vi "ke37xx Open Channels.vi"(0 "VISA Resource Name":refnum<visa-resource-name>, 1 "Channel List":string, 7 "Open All (False)":bool, 11 "error in (no error)":errorcluster) -> (4 "VISA Resource Name Out":refnum<visa-resource-name>, 15 "error out":errorcluster)   [LabVIEW 2009, in "Keithley 3700 Series.lvlib"]
doc: "This VI allows you to open a series of channels or to open all channels."
uses:
  <instrlib>/Keithley 3706/Keithley 3700 Series.lvlib
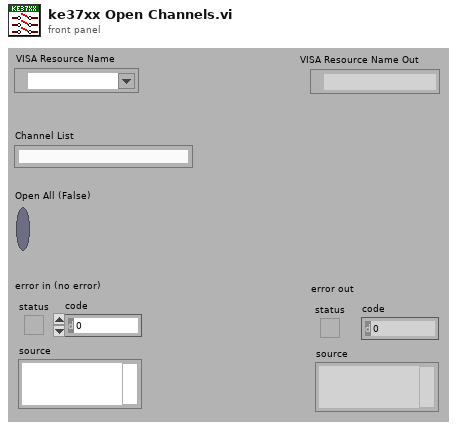
[diagram p1: front panel]
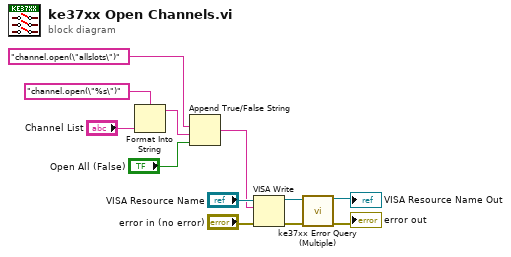
[diagram p0: block diagram]
diagram:
  n1 = Format Into String(format string="channel.open(\"%s\")", "Channel List") -> (resulting string=w2:string)  [unwired: 2 in, 1 out]
  n2 = Append True/False String(1:"Open All (False)", 2:w2, 3:"channel.open(\"allslots\")") -> (0:w1:string)  [unwired: 1 out]
  n3 = VISA Write(VISA resource name="VISA Resource Name", write buffer=w1, error in (no error)="error in (no error)") -> (VISA resource name out=w9:refnum<visa-resource-name>, error out=w7:errorcluster)  [unwired: 1 out]
  n4 = call <instrlib>:"ke37xx Error Query (Multiple).vi"("VISA resource name"=w9, "error in (no error)"=w7) -> ("VISA resource name out"=→"VISA Resource Name Out":refnum<visa-resource-name>, "error out"=→"error out":errorcluster)  [unwired: 12 out]
